vi "Untitled 3.vi"() -> ()   [LabVIEW 2016]
panel:
  in  "Length":dbl
  in  "Resistivity":dbl
  out "Numeric":dbl
  in  "AWG":dbl
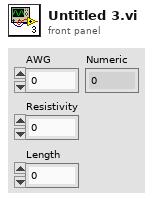
[diagram p1: front panel]
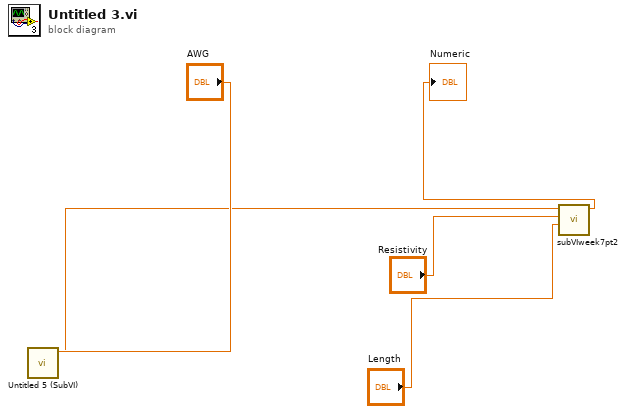
[diagram p0: block diagram]
diagram:
  n1 = call "Untitled 5 (SubVI)"("AWG"="AWG") -> ("Numeric"=w2:dbl)  [unwired: 10 in]
  n2 = call "subVIweek7pt2.vi"("Length"="Length", "Resistivity"="Resistivity", "Numeric in"=w2) -> ("Numeric out"=→"Numeric":dbl)  [unwired: 8 in]
